vi "List Index&Feed.vi"(8 "error in (no error)":errorcluster, 11 "Artifactory.VIPM in":refnum<class "Artifactory.VIPM.lvclass">) -> (0 "error out":errorcluster, 2 "Index & Feed":string[](array[string]), 3 "Artifactory.VIPM out":refnum<class "Artifactory.VIPM.lvclass">)   [LabVIEW 2021, in "Artifactory.VIPM.lvclass"]
uses:
  Artifactory.VIPM.lvclass
  C:/Repositories/LVOS/Artifactory/lv-src/Artifactory/Artifactory.lvclass
  Artifactory/Artifactory.lvclass
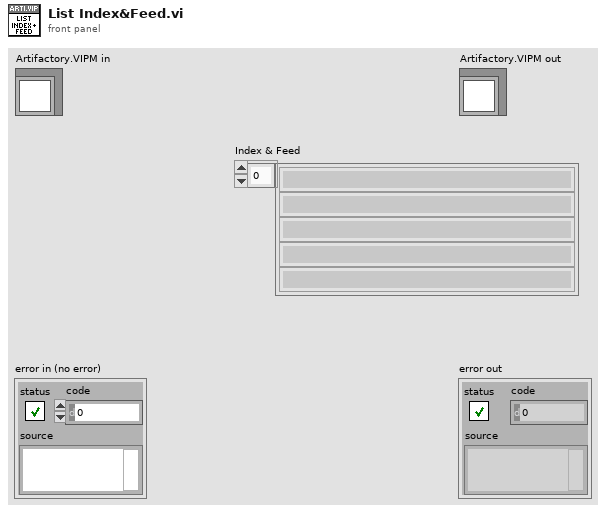
[diagram p1: front panel]
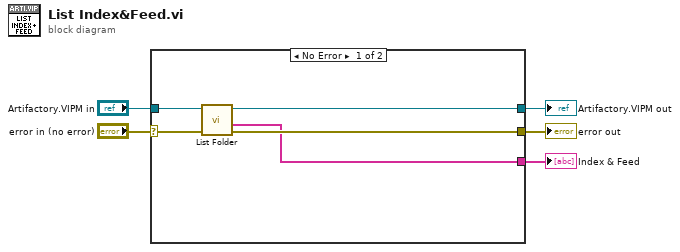
[diagram p0: block diagram]
diagram:
  n1 = case shown="No Error" "error in (no error)" {
    selector: "error in (no error)" -> [w8 w12]
    tunnel: [w7 w12] -> w4
    tunnel: [w10 w11] -> w2
    tunnel: "Artifactory.VIPM in" -> [w9 w11]
    tunnel: [w6 _] -> w1
    frame No Error {
      n2 = call "List Folder.vi"("error in (no error)"=w8, "Artifactory in"=w9) -> ("error out"=w7:errorcluster, "Files"=w6:string[], "Artifactory out"=w10:refnum<class "Artifactory.VIPM.lvclass">)  [unwired: 6 in, 1 out]
    }
    frame Error {
    }
  }
  "error out" <- w4
  "Artifactory.VIPM out" <- w2
  "Index & Feed" <- w1
